vi "Defend.vi"(11 "AI Manager in":refnum<class "AI Manager.lvclass">) -> (2 "Direction out":cluster{dbl, dbl}, 5 "Boost ?":bool)   [LabVIEW 2024, in "AI Manager.lvclass"]
doc: "MIT Licence\nCopyright (c) 2024 David Grollier"
uses:
  AI Manager.lvclass
  AI Manager.lvclass/AI Manager.ctl
  Game Componants/Game Board Component/Movable/Movable.lvclass/Movable.ctl
  Game Componants/Game Componants.lvclass/Game Componants.ctl
  <vilib>/Analysis/_algsub.llb/Vector Norm.vi
  <vilib>/Analysis/_algsub.llb/Real Vector Norm.vi
  Game Componants/Game Board Component/Movable/Flying Saucer/Flying Saucer.lvclass
  Game Componants/Game Board Component/Movable/Movable.lvclass
  Utils/Utils.lvlib
  Game Componants/Game Componants.lvclass
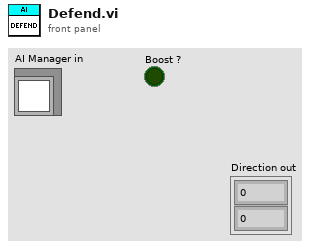
[diagram p1: front panel]
types:
  T1 = typedef "Coordinates.ctl" = cluster{"x":dbl, "y":dbl}
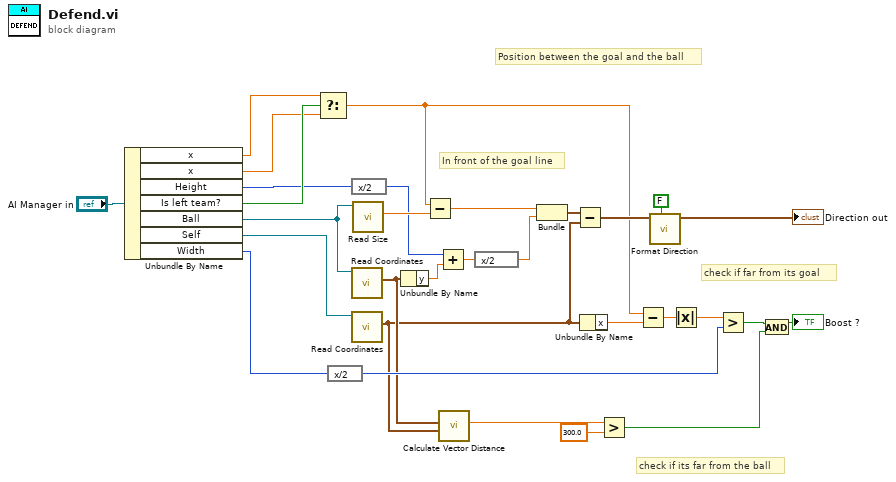
[diagram p0: block diagram]
diagram:
  # "check if its far from the ball"
  # "check if far from its goal"
  # "In front of the goal line"
  # "Position between the goal and the ball"
  n1 = Unbundle By Name("AI Manager in") -> ("x"=w13:dbl, "x"=w14:dbl, "Height"=w10:u32, "Is left team?"=w15:bool, "Ball"=w22:refnum<class "Movable.lvclass">, "Self"=w24:refnum<class "Flying Saucer.lvclass">, "Width"=w8:u32)
  n2 = Select(t=w13, s=w15, f=w14) -> (s? t:f=w12:dbl)
  n3 = expression code="x/2"(w8) -> (w7:u32)
  n4 = expression code="x/2"(w10) -> (w9:u32)
  n5 = call "Read Coordinates.vi"("Game Componants in"=w22) -> ("Coordinates"=w6:T1)  [unwired: 10 in]
  n6 = call "Read Coordinates.vi"("Game Componants in"=w24) -> ("Coordinates"=w5:T1)  [unwired: 10 in]
  n7 = call "Read Size.vi"("Movable in"=w22) -> ("Size"=w21:dbl)  [unwired: 10 in]
  n8 = Unbundle By Name(w6) -> ("y"=w23:dbl)
  n9 = Subtract(x=w12, y=w21) -> (x-y=w20:dbl)
  n10 = Add(x=w9, y=w23) -> (x+y=w19:dbl)
  n11 = call "Calculate Vector Distance.vi"("V2"=w5, "V1"=w6) -> ("Distance out"=w4:dbl)  [unwired: 9 in]
  n12 = expression code="x/2"(w19) -> (w28:dbl)
  n13 = Bundle(w20, w28) -> (w27:cluster{dbl, dbl})  [unwired: 1 in]
  n14 = Subtract(x=w27, y=w5) -> (x-y=w26:T1)
  n15 = Unbundle By Name(w5) -> ("x"=w18:dbl)
  n16 = Greater?(x=w4, y=300.0) -> (0:w1:bool)
  n17 = Subtract(x=w12, y=w18) -> (x-y=w17:dbl)
  n18 = call "Format Direction.vi"("Xbox Controller (T)"=FALSE ("Analog Stick? (T)"), "Direction in"=w26) -> ("Formated Direction out"=→"Direction out":cluster{dbl, dbl})  [unwired: 9 in]
  n19 = Absolute Value(x=w17) -> (abs(x)=w11:dbl)
  n20 = Greater?(x=w11, y=w7) -> (0:w16:bool)
  n21 = And(x=w16, y=w1) -> (x .and. y?=→"Boost ?":bool)
